vi "set_up_histogramming.vi"(8 "error in (no error)":errorcluster, 11 "swabian_local_data 2":T1={"events"={"update_status"=refnum, "update_chart"=refnum, "update_xy"=refnum, "send_channel_data"=refnum}, "stop_q"=refnum, "tagger_reference"=refnum, "connect_button"=refnum, "counter_reference"=refnum, "tagger_stream_reference"=refnum, "log_reference"=refnum, "current_log_offset"=0, "tt20_buffer_q"=refnum, "stream_to_file_button"=refnum, "num_records"=0, "connected?"=FALSE, "plots"=refnum, "histogram_bin_edges"=[], "histogrammer"=refnum, "plot_lifetimes"=refnum, "xy_graph"=refnum, "Reference\nChannel"=enum."ch0", "trigger_channels"=[], "filter_channels"=[], "active_channels"=[], "acq_mode"=0, "Reference\nChannel"=enum."ch0", "acq_time"=0, "sync_period_ps"=0, "raw_stream_path"=path "", "Leftovers"={"missing_sync_data"=[], "missing_events"=0}, "first_batch"=0, "first_sync_stamp"=0, "lifetime_settings"={"Plot Lifetimes"=FALSE, "start_time"=0.0, "stop_time"=0.0, "n_bins"=0}, "Histogram_bins"=[], "last_processed_data"=[], "histogram_data"=[]}) -> (0 "error out":errorcluster, 2 "chart_counts?":bool, 3 "swabian_local_data 3":T1={"events"={"update_status"=refnum, "update_chart"=refnum, "update_xy"=refnum, "send_channel_data"=refnum}, "stop_q"=refnum, "tagger_reference"=refnum, "connect_button"=refnum, "counter_reference"=refnum, "tagger_stream_reference"=refnum, "log_reference"=refnum, "current_log_offset"=0, "tt20_buffer_q"=refnum, "stream_to_file_button"=refnum, "num_records"=0, "connected?"=FALSE, "plots"=refnum, "histogram_bin_edges"=[], "histogrammer"=refnum, "plot_lifetimes"=refnum, "xy_graph"=refnum, "Reference\nChannel"=enum."ch0", "trigger_channels"=[], "filter_channels"=[], "active_channels"=[], "acq_mode"=0, "Reference\nChannel"=enum."ch0", "acq_time"=0, "sync_period_ps"=0, "raw_stream_path"=path "", "Leftovers"={"missing_sync_data"=[], "missing_events"=0}, "first_batch"=0, "first_sync_stamp"=0, "lifetime_settings"={"Plot Lifetimes"=FALSE, "start_time"=0.0, "stop_time"=0.0, "n_bins"=0}, "Histogram_bins"=[], "last_processed_data"=[], "histogram_data"=[]})   [LabVIEW 2018]
uses:
  swabian_local_data_tdef.ctl
  swabian_events_tdef.ctl
  update_chart_tdef.ctl
  channel_data_tdef.ctl
  C:/Users/bspoka/Documents/swabian_LV/lib/TTCSharp32.dll
  lib/TTCSharp32.dll
  swabian_buffer_tdef.ctl
  reference_checkbox_tdef.ctl
  lifetime_settings.ctl
  <vilib>/Analysis/1siggen.llb/Ramp Pattern by Samples.vi
  <vilib>/Analysis/NI_AALBase.lvlib
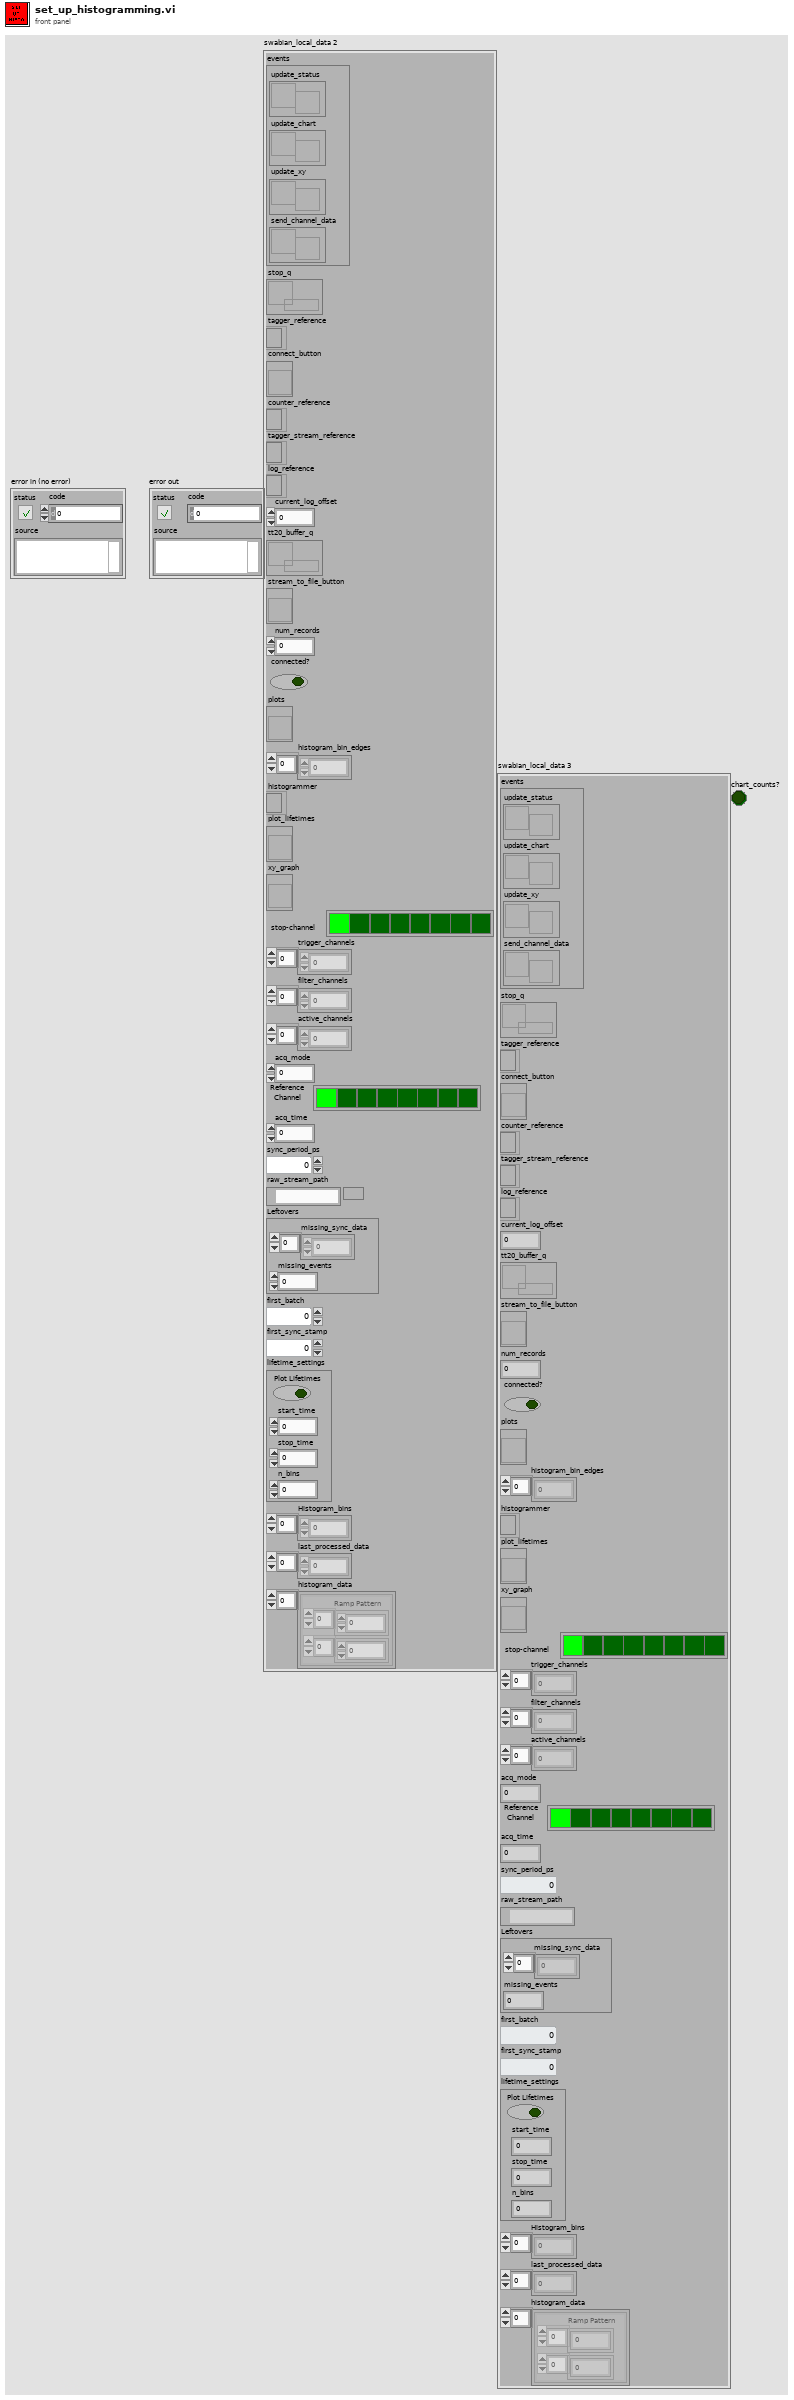
[diagram p1: front panel]
types:
  T1 = typedef "swabian_local_data_tdef.ctl" = cluster{"events":T2, "stop_q":refnum<queue>, "tagger_reference":refnum<k24>, "connect_button":refnum<vi>, "counter_reference":refnum<k24>, "tagger_stream_reference":refnum<k24>, "log_reference":refnum<file>, "current_log_offset":i64, "tt20_buffer_q":refnum<queue>, "stream_to_file_button":refnum<vi>, "num_records":u64, "connected?":bool, "plots":refnum<vi>, "histogram_bin_edges":i64[], "histogrammer":refnum<k24>, "plot_lifetimes":refnum<vi>, "xy_graph":refnum<vi>, "Reference\nChannel":T3, "trigger_channels":i32[], "filter_channels":i32[], "active_channels":i32[], "acq_mode":i32, "Reference\nChannel":T3, "acq_time":i64, "sync_period_ps":i64, "raw_stream_path":path, "Leftovers":cluster{"missing_sync_data":i64[], "missing_events":i32}, "first_batch":i32, "first_sync_stamp":i64, "lifetime_settings":T4, "Histogram_bins":dbl[], "last_processed_data":i64[], "histogram_data":cluster{"Ramp Pattern":dbl[], dbl[]}[]}
  T2 = typedef "swabian_events_tdef.ctl" = cluster{"update_status":refnum<user-event>, "update_chart":refnum<user-event>, "update_xy":refnum<user-event>, "send_channel_data":refnum<user-event>}
  T3 = typedef "reference_checkbox_tdef.ctl" = enum32{"No Selection", "ch0", "ch1", "ch2", "ch3", "ch4", "ch5", "ch6", "ch7"}
  T4 = typedef "lifetime_settings.ctl" = cluster{"Plot Lifetimes":bool, "start_time":dbl, "stop_time":dbl, "n_bins":i32}
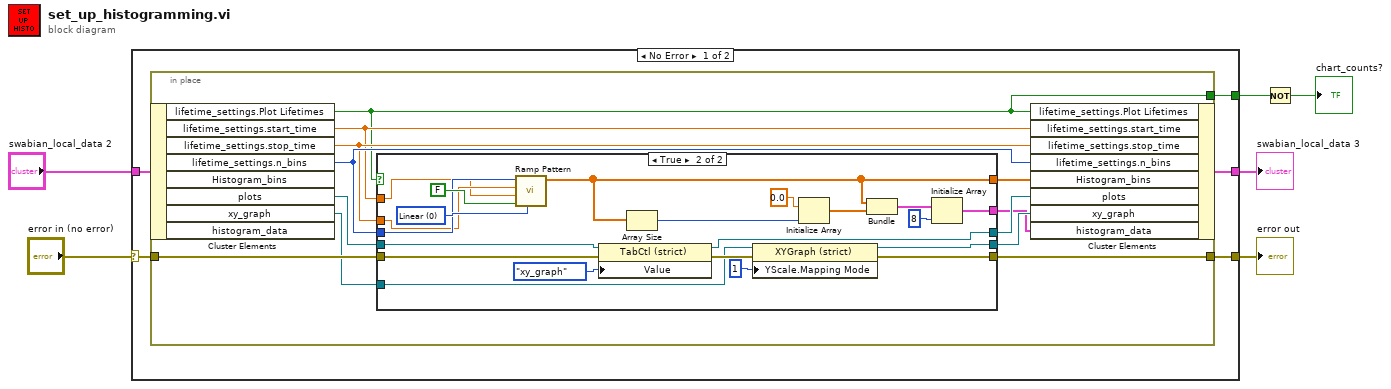
[diagram p0: block diagram]
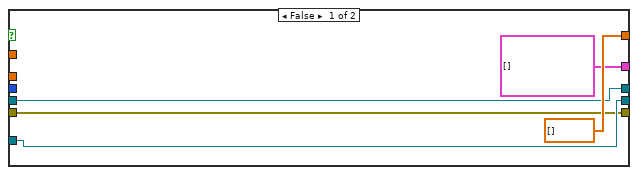
[diagram p2: hidden frame]
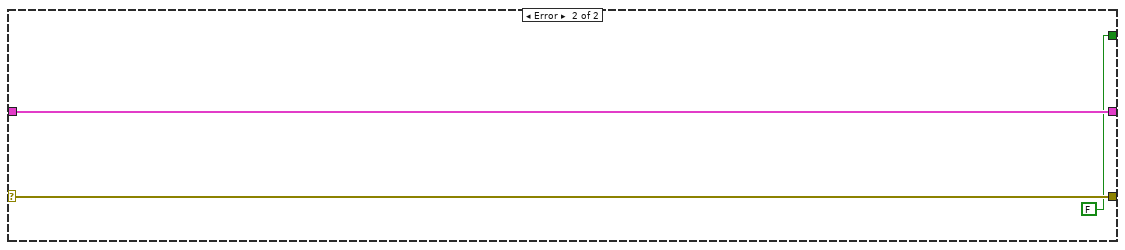
[diagram p3: hidden frame]
diagram:
  n1 = case shown="No Error" "error in (no error)" {
    selector: "error in (no error)" -> [w10 w52]
    tunnel: "swabian_local_data 2" -> [w11 w51]
    tunnel: [w9 w52] -> w4
    tunnel: [w8 w51] -> w3
    tunnel: [w7 FALSE] -> w2
    frame No Error {
      n2 = in-place {
        in-place-border: w10 -> [w17]
        in-place-border: [w13] -> w9
        in-place-border: [w14] -> w7
        n3 = in-place-cluster #1(w11) -> ("lifetime_settings.Plot Lifetimes"=w14:bool, "lifetime_settings.start_time"=w20:dbl, "lifetime_settings.stop_time"=w21:dbl, "lifetime_settings.n_bins"=w22:i32, "plots"=w19:refnum<vi>, "xy_graph"=w16:refnum<vi>)  [unwired: 2 out]
        n4 = case shown="True" w14 {
          tunnel: [dbl[] [] ("Ramp Pattern") w35] -> w23
          tunnel: w22 -> [_ w47]
          tunnel: w21 -> [_ w46]
          tunnel: w20 -> [_ w45]
          tunnel: w19 -> [w26 w44]
          tunnel: [w26 w42] -> w18
          tunnel: w17 -> [w25 w41]
          tunnel: w16 -> [w27 w39]
          tunnel: [w27 w37] -> w15
          tunnel: [w25 w36] -> w13
          tunnel: [cluster{"Ramp Pattern":dbl[], dbl[]}[] [] w29] -> w12
          frame False {
          }
          frame True {
            w49 = u16 0 items=["Linear", "Logarithmic"] ("type")
            n5 = call-poly <vilib>:"Ramp Pattern.vi"("type"=w49, "exclude end?"=FALSE, "start"=w45, "end"=w46, "samples"=w47) -> ("Ramp Pattern"=w35:dbl[])  [unwired: 5 in, 1 out]
            n6 = property class="TabCtl (strict)"(reference=w44, error in=w41, "Value"=enum32{"chart", "xy_graph"}."xy_graph") -> (reference out=w42:refnum<vi>, error out=w40:errorcluster)
            n7 = Array Size(array=w35) -> (size(s)=w34:i32)
            n8 = property class="XYGraph (strict)"(reference=w39, error in=w40, "YScale.Mapping Mode"=u8 1 ("Y Scale.Mapping Mode")) -> (reference out=w37:refnum<vi>, error out=w36:errorcluster)
            n9 = Initialize Array(0.0 ("element"), w34) -> (w32:dbl[])
            n10 = Bundle("Ramp Pattern"=w35, w32) -> (w31:cluster{"Ramp Pattern":dbl[], dbl[]})  [unwired: 1 in]
            n11 = Initialize Array(w31, 8 ("dimension size")) -> (w29:cluster{"Ramp Pattern":dbl[], dbl[]}[])
          }
        }
        n12 = in-place-cluster #1("lifetime_settings.Plot Lifetimes"=w14, "lifetime_settings.start_time"=w20, "lifetime_settings.stop_time"=w21, "lifetime_settings.n_bins"=w22, "Histogram_bins"=w23, "plots"=w18, "xy_graph"=w15, "histogram_data"=w12) -> (w8:T1)
      }
    }
    frame Error {
    }
  }
  "error out" <- w4
  "swabian_local_data 3" <- w3
  n13 = Not(x=w2) -> (.not. x?=→"chart_counts?":bool)
